vi "Set Limits.vi"(8 "error in (no error)":errorcluster, 9 "?":T1(array[cluster]) {"stimulus (Hz,dB,s)" format="%.2e"; "limit type" items=["sloping line", "flat line", "single point"]; "lower/delta (dB,degrees,units)" format="%.2e"; "upper/middle (dB,degrees,units)" format="%.2e"}, 11 "VISA resource name":refnum<visa-resource-name>) -> (0 "error out":errorcluster, 3 "VISA resource name out":refnum<visa-resource-name>)   [LabVIEW 2018, in "Agilent 87XX Series.lvlib"]
doc: "This VI for the HP8753B Network Analyzer is used for setting limit tests. Limits are set the same way as they are set from the instrument itself. The one difference is that you must throw a switch to control if limits are set by their upper and lower values or by their middle and delta values."
uses:
  Agilent 87XX Series.lvlib
panel:
  # "upper/lower"
  # "middle/delta"
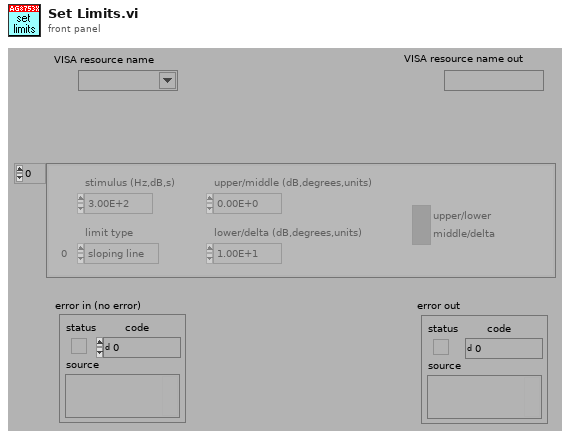
[diagram p1: front panel]
types:
  T1 = cluster{bool, "stimulus (Hz,dB,s)":dbl, "upper/middle (dB,degrees,units)":dbl, "lower/delta (dB,degrees,units)":dbl, "limit type":u16}[]
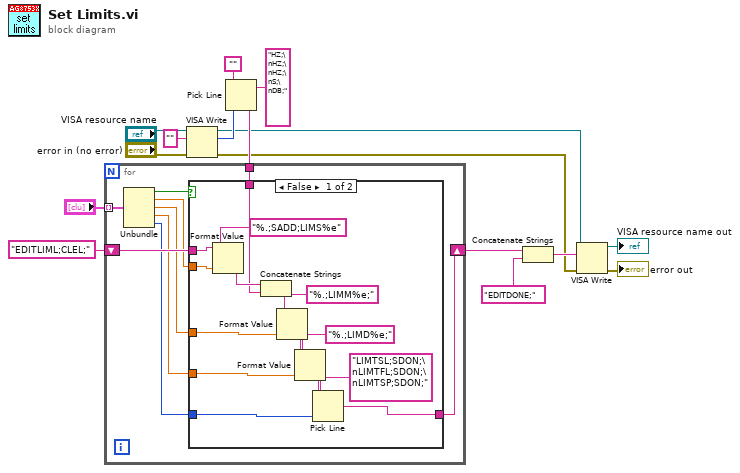
[diagram p0: block diagram]
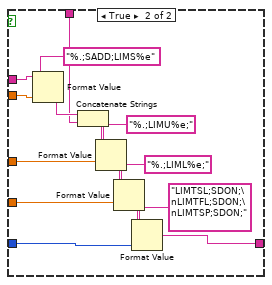
[diagram p2: hidden frame]
diagram:
  n1 = VISA Write(VISA resource name="VISA resource name", write buffer="", error in (no error)="error in (no error)") -> (VISA resource name out=w4:refnum<visa-resource-name>, return count=w9:u32, error out=w3:errorcluster)
  n2 = Pick Line(string ("")="", multi-line string="HZ;\nHZ;\nHZ;\nS;\nDB;", line index=w9) -> (output string=w10:string)
  n3 = for {
    tunnel: "?" -> [w25] mode=indexing
    shift-right: [w18] -> w15
    shift-left: "EDITLIML;CLEL;" -> [w24]
    tunnel: w10 -> [w17]
    n4 = Unbundle(w25) -> (w22:bool, "stimulus (Hz,dB,s)"=w21:dbl, "upper/middle (dB,degrees,units)"=w20:dbl, "lower/delta (dB,degrees,units)"=w19:dbl, "limit type"=w23:u16)
    n5 = case shown="False" w22 {
      tunnel: w24 -> [w40 w55]
      tunnel: w21 -> [w33 w47]
      tunnel: w20 -> [w32 w46]
      tunnel: w19 -> [w31 w45]
      tunnel: w23 -> [w30 w44]
      tunnel: [w29 w43] -> w18
      tunnel: w17 -> [w27 w42]
      frame False {
        n6 = Format Value(string ("")=w40, format string="%.;SADD;LIMS%e", value (0)=w33) -> (output string=w28:string)
        n7 = Concatenate Strings(w28, w27) -> (w26:string)
        n8 = Format Value(string ("")=w26, format string="%.;LIMM%e;", value (0)=w32) -> (output string=w36:string)
        n9 = Format Value(string ("")=w36, format string="%.;LIMD%e;", value (0)=w31) -> (output string=w34:string)
        n10 = Pick Line(string ("")=w34, multi-line string="LIMTSL;SDON;\nLIMTFL;SDON;\nLIMTSP;SDON;", line index=w30) -> (output string=w29:string)
      }
      frame True {
        n11 = Format Value(string ("")=w55, format string="%.;SADD;LIMS%e", value (0)=w47) -> (output string=w52:string)
        n12 = Concatenate Strings(w52, w42) -> (w41:string)
        n13 = Format Value(string ("")=w41, format string="%.;LIMU%e;", value (0)=w46) -> (output string=w50:string)
        n14 = Format Value(string ("")=w50, format string="%.;LIML%e;", value (0)=w45) -> (output string=w48:string)
        n15 = Format Value(string ("")=w48, format string="LIMTSL;SDON;\nLIMTFL;SDON;\nLIMTSP;SDON;", value (0)=w44) -> (output string=w43:string)
      }
    }
  }
  n16 = Concatenate Strings(w15, "EDITDONE;") -> (w14:string)
  n17 = VISA Write(VISA resource name=w4, write buffer=w14, error in (no error)=w3) -> (VISA resource name out=→"VISA resource name out":refnum<visa-resource-name>, error out=→"error out":errorcluster)  [unwired: 1 out]
